vi "Multi_OUI_NON.vi"(8 "errin":errorcluster caption="entrée d'erreur (pas d'erreur)", 9 "errinb":bool, 10 "Tableau":string[](array[string])) -> (0 "errout":errorcluster caption="sortie d'erreur", 3 "isok?":bool)   [LabVIEW 2020]
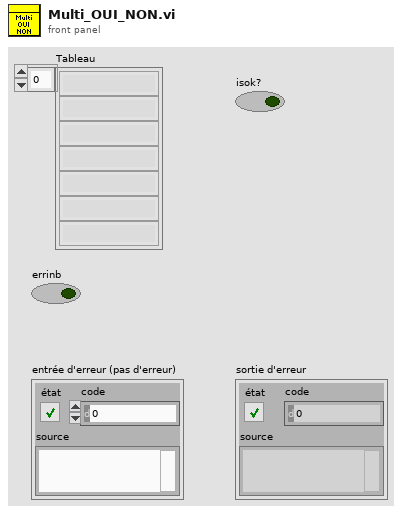
[diagram p1: front panel]
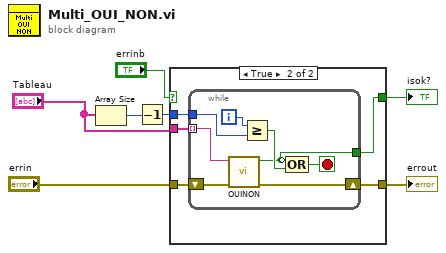
[diagram p0: block diagram]
diagram:
  n1 = Array Size(array="Tableau") -> (size(s)=w2:i32)
  n2 = Decrement(x=w2) -> (x-1=w1:i32)
  n3 = case shown="True" "errinb" {
    selector: "errinb" -> [w8 _]
    tunnel: "Tableau" -> [_ w14]
    tunnel: w1 -> [_ w13]
    tunnel: [w8 w12] -> w4
    tunnel: [w9 w11] -> w5
    tunnel: "errin" -> [w9 w10]
    frame False {
    }
    frame True {
      n4 = while {
        tunnel: w14 -> [w20] mode=indexing
        tunnel: w13 -> [w21]
        shift-right: [w18] -> w11
        shift-left: w10 -> [w19]
        tunnel: [w15] -> w12
        i -> [w22]
        stop <- w16 stop-if-true
        n5 = call "OUINON.vi"("errin"=w19, "image"=w20) -> ("error out"=w18:errorcluster, "OUI/NON"=w15:bool)  [unwired: 8 in]
        n6 = Greater Or Equal?(x=w22, y=w21) -> (x >= y?=w17:bool)
        n7 = Compound Arithmetic op=OR ("Opérateur arithmétique")(invert w15, w17) -> (w16:bool)
      }
    }
  }
  "errout" <- w5
  "isok?" <- w4
